vi "Convert State String to Enum.vi"(9 "state in":string, 12 "error in":errorcluster) -> (10 "state out":T1, 14 "error out":errorcluster)   [LabVIEW 2015, in "TLB` Template.lvlib" / "{TMPL} TLB`.lvclass"]
doc: "Convert string to State.ctl enum.\n\n<B>Input Parameters</B>\n\n<B>state in</B> is the current state of the system of type string.\n\n<B>error in</B> describes error conditions that occur before this node runs. This input provides standard error in functionality.\n\n<B>Output Parameters</B>\n\n<B>state out</B> is the current state of the system of type enum.\n\n<B>error out</B> contains error information. This output provides standard error out functionality."
uses:
  {TMPL} TLB`.lvclass
  State Machine/State.ctl
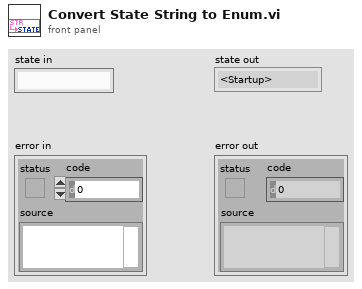
[diagram p1: front panel]
types:
  T1 = typedef "TLB` Template.lvlib/{TMPL} TLB`.lvclass/State.ctl" = enum16{"<Startup>", "Idle", "<Shutdown>", "<Error>"}
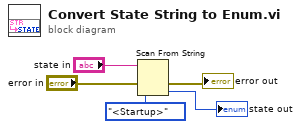
[diagram p0: block diagram]
diagram:
  n1 = Scan From String(input string="state in", error in="error in", default 1=State."<Startup>" ("State")) -> (error out=→"error out":errorcluster, output 1=→"state out":T1)  [unwired: 2 in, 2 out]
